vi "UPRcontroller_v00_basedonlsmv66.vi"() -> ()   [LabVIEW 2015] (continued)
                        n4087 = call "tt_timeandsamples.vi"("bin"=w857, "refreshtime"=w851, "srateAODOtt"=w854, "tot#ofsamples"=w859) -> ("refreshrate"=w855:dbl, "refreshbuffer"=w856:i32, "timetracecycles"=w861:i32)  [unwired: 5 in]
                        n4088 = local read "bin"() -> (w858:dbl)
                        n4089 = call "2pparameters.vi"("command"="get") -> ("params out"=w870:T12)  [unwired: 1 in]
                        n4090 = Bundle By Name(cluster=w870, "Drawing Mode"=w843, "measpoints"=w859, "tt_cycles"=w861, "refreshbuffer"=w856, "refreshrate"=w855, "Vx-ref"=w862, "Vy-ref"=w864, "srate"=w853, "finite"=w866, "cont"=w865, "wavdet"=w867, "avpp"=w863, "srateAODO"=w860, "bufferAI"=w856, "bin"=w858, "Angle Img"=w850, "Vxminref"=w849, "Vxmaxref"=w848, "Vyminref"=w847, "Vymaxref"=w846, "Xpixels Img"=w845, "Ypixels Img"=w844, "Pel"=w842, "Vz-reset"=0.0, "AIoverride"=w840, "type"="Timetrace") -> (w868:T12)
                        n4091 = Reciprocal(x=w855) -> (1/x=w852:dbl)
                        n4092 = local write "refreshtime"(w852) -> ()
                        n4093 = call "2pparameters.vi"("Params in"=w868, "command"="set") -> ()  [unwired: 1 out]
                      }
                      frame "Lifetime (point)" {
                      }
                    }
                  }
                  frame #1 {
                    w873 = FALSE ("wavdet")
                    n4094 = call "2pparameters.vi"("command"="get") -> ("params out"=w877:T12)  [unwired: 1 in]
                    n4095 = Bundle By Name(cluster=w877, "finite"=w873, "cont"=w873, "wavdet"=TRUE) -> (w874:T12)
                    n4096 = call "2pparameters.vi"("Params in"=w874, "command"="set") -> ()  [unwired: 1 out]
                  }
                  frame #2 {
                    n4097 = local read "DO channels"() -> (w885:u16)
                    n4098 = call "2pparameters.vi"("command"="get") -> ("params out"=w883:T12)  [unwired: 1 in]
                    n4099 = in-place {
                      in-place-border: w885 -> [w890]
                      in-place-border: [w887] -> w880
                      in-place-border: [w886] -> w879
                      n4100 = in-place-cluster #52(w883) -> ("aDO"=w889:u32[])
                      n4101 = call "remove channel from active arrayv2.vi"("line array in"=w889, "line to remove"=w890) -> ("line array out"=w888:u32[], "removal"=w887:bool, "index"=w886:i32)
                      n4102 = in-place-cluster #52("aDO"=w888) -> (w881:T12)
                    }
                    n4103 = local write "remDO"(w880) -> ()
                    n4104 = call "2pparameters.vi"("Params in"=w881, "command"="set") -> ()  [unwired: 1 out]
                  }
                  frame #3 {
                    n4105 = local read "remDO"() -> (w891:bool)
                    n4106 = case shown="True" w891 {
                      frame False {
                      }
                      frame True {
                        n4107 = call "Used AO lines.vi"() -> ("used AO names"=w895:string[], "used AO lines"=w897:tag[])  [unwired: 2 in]
                        n4108 = local write "Analog Used Lines"(w897) -> ()
                        n4109 = local write "Analog Used Names"(w895) -> ()
                        n4110 = call "Used DO lines.vi"() -> ("used DO names"=w893:string[], "used DO lines"=w892:tag[])  [unwired: 2 in]
                        n4111 = control-ref of="Analog Lines Plot"() -> (w896:refnum<vi>)
                        n4112 = control-ref of="Digital Lines Plot"() -> (w894:refnum<vi>)
                        n4113 = local write "Digital Used Lines"(w892) -> ()
                        n4114 = local write "Digital Used Names"(w893) -> ()
                        n4115 = call "prepAOWaveplot.vi"("WaveformGraph in"=w896, "Analog Used Names"=w895) -> ()  [unwired: 1 in]
                        n4116 = call "prepDOWaveplot.vi"("DigitalGraph in"=w894, "used DO names"=w893) -> ()  [unwired: 1 in]
                      }
                    }
                  }
                  frame #4 {
                    n4117 = local read "remDO"() -> (w899:bool)
                    n4118 = case shown="True" w899 {
                      tunnel: w898 -> [_ w900]
                      frame False {
                      }
                      frame True {
                        n4119 = call "waveformparamsv2.vi"("command"="rem DO", "index"=w900) -> ()  [unwired: 3 in, 3 out]
                      }
                    }
                  }
                  frame #5 {
                    n4120 = local read "Meastab"() -> (w905:enum32{"X-Y Image", "Linescan", "Timetrace"})
                    n4121 = property on="refwf" class="Ring (strict)"() -> ("RingText.Text"=w912:string)  [unwired: 2 in, 2 out]
                    n4122 = call "waveformsDObuffer.vi"("command"="get") -> ("DO wf out"=w911:digitalwaveform[])  [unwired: 1 in]
                    n4123 = case shown="\"Timetrace\"" w905 {
                      tunnel: [w921 w922] -> w904
                      frame "X-Y Image", Default {
                        n4124 = local read "Sampling rate"() -> (w921:dbl)
                      }
                      frame "Timetrace" {
                        n4125 = local read "srateAODOtt"() -> (w922:dbl)
                      }
                    }
                    n4126 = call "waveformsAObuffer.vi"("command"="get") -> ("AO wf out"=w920:waveform(dbl)[])  [unwired: 1 in]
                    n4127 = Delete From Array(array=w911, length=1, index=w909) -> (array with subset deleted=w908:digitalwaveform[])  [unwired: 1 out]
                    n4128 = call "correctwaveformsizetemp.vi"("new sampling frequency (Hz)"=w904, "start"=FALSE, "reference waveforms to"=w912, "Analog waveforms in"=w920, "stop"=FALSE, "Digital waveforms in"=w908) -> ("analog wf out"=w915:waveform(dbl)[], "Digital wf out"=w913:digitalwaveform[], "measpoints"=w906:i32)
                    n4129 = local read "wavdet"() -> (w907:bool)
                    n4130 = call "waveformsAObuffer.vi"("AO wf in"=w915, "command"="set") -> ()  [unwired: 1 out]
                    n4131 = call "waveformsDObuffer.vi"("DO wf in"=w913, "command"="set") -> ()  [unwired: 1 out]
                    n4132 = local write "Analog Lines Plot"(w915) -> ()
                    n4133 = local write "Digital Lines Plot"(w913) -> ()
                    n4134 = call "GetNumCamFramesv2.vi"("Digital Waveform Graph"=w913) -> ("Numeric"=w914:i32)  [unwired: 10 in]
                    n4135 = case shown="True" w907 {
                      tunnel: w906 -> [_ w923]
                      frame False {
                      }
                      frame True {
                        n4136 = local write "# of frames"(w923) -> ()
                      }
                    }
                    n4137 = local write "Total Camera Frames"(w914) -> ()
                  }
                  frame #6 {
                    w924 = FALSE ("addAO")
                    n4138 = local read "finite samples"() -> (w925:bool)
                    n4139 = local read "continuous"() -> (w926:bool)
                    n4140 = local read "wavdet"() -> (w927:bool)
                    n4141 = local write "remDO"(w924) -> ()
                    n4142 = call "2pparameters.vi"("command"="get") -> ("params out"=w930:T12)  [unwired: 1 in]
                    n4143 = Bundle By Name(cluster=w930, "finite"=w925, "cont"=w926, "wavdet"=w927) -> (w928:T12)
                    n4144 = property on="Rem DO wave" class="Bool (strict)"("Val(Sgnl)"=w924) -> ()  [unwired: 2 in, 2 out]
                    n4145 = call "2pparameters.vi"("Params in"=w928, "command"="set") -> ()  [unwired: 1 out]
                  }
                }
              }
            }
          }
          event "load changed DO wave": Value Change {
            n4146 = event-data() -> ("NewVal"=w932:bool)  [unwired: 1 in, 5 out]
            n4147 = case shown="True" w932 {
              frame False {
              }
              frame True {
                n4148 = stacked-sequence {
                  seq-local: [_ _ w1040 _ _] -> [_ _ _ w1057 _]
                  seq-local: [_ _ w1039 _ _] -> [_ _ _ w1056 _]
                  frame #0 {
                    n4149 = local read "Measurement"() -> (w934:T4)
                    n4150 = local write "changeDO"(TRUE ("addAO")) -> ()
                    n4151 = case shown="\"X-Y-t movie\", Default" w934 {
                      frame "X-Y-t movie", Default {
                        n4152 = local read "avpp"() -> (w955:i32)
                        n4153 = local read "Angle ref"() -> (w954:dbl)
                        n4154 = local read "ROI Type"() -> (w953:u16)
                        n4155 = local read "xpixels ref"() -> (w950:i32)
                        n4156 = local read "Vx-min ref"() -> (w949:dbl)
                        n4157 = local read "Vx-max ref"() -> (w948:dbl)
                        n4158 = local read "ypixels ref"() -> (w946:i32)
                        n4159 = local read "Vy-min ref"() -> (w947:dbl)
                        n4160 = local read "Vy-max ref"() -> (w943:dbl)
                        n4161 = local read "Sampling rate"() -> (w937:dbl)
                        n4162 = local read "finite samples"() -> (w938:bool)
                        n4163 = local read "continuous"() -> (w941:bool)
                        n4164 = local read "wavdet"() -> (w942:bool)
                        n4165 = local read "# of frames"() -> (w940:i32)
                        n4166 = local read "maxbufferAI"() -> (w939:i32)
                        n4167 = local read "Override AI buffer"() -> (w935:bool)
                        n4168 = call "2pparameters.vi"("command"="get") -> ("params out"=w952:T12)  [unwired: 1 in]
                        n4169 = Bundle By Name(cluster=w952, "type"="X-Y-t movie", "avpp"=w955, "Angle Img"=w954, "Xpixels Img"=w950, "Vx-min Img"=w949, "VX-max Img"=w948, "Ypixels Img"=w946, "Vy-min Img"=w947, "Vy-max Img"=w943, "srate"=w937, "srate Img"=w937, "finite"=w938, "cont"=w941, "wavdet"=w942, "measpoints"=w940, "maxbufferAI"=w939, "Drawing Mode"=w953, "Vz-reset"=0.0, "AIoverride"=w935) -> (w944:T12)
                        n4170 = call "2pparameters.vi"("Params in"=w944, "command"="set") -> ()  [unwired: 1 out]
                      }
                      frame "X-Y-Z stack" {
                        n4171 = call "2pparameters.vi"("command"="get") -> ("params out"=w959:T12)  [unwired: 1 in]
                        n4172 = Bundle By Name(cluster=w959, "type"="X-Y-Z stack") -> (w957:T12)
                        n4173 = call "2pparameters.vi"("Params in"=w957, "command"="set") -> ()  [unwired: 1 out]
                      }
                      frame "Lifetime (scan)" {
                        n4174 = call "2pparameters.vi"("command"="get") -> ("params out"=w964:T12)  [unwired: 1 in]
                        n4175 = Bundle By Name(cluster=w964, "type"="Lifetime (scan)") -> (w962:T12)
                        n4176 = call "2pparameters.vi"("Params in"=w962, "command"="set") -> ()  [unwired: 1 out]
                      }
                      frame "Lifetime (contour)" {
                        n4177 = local read "Vy-min draw"() -> (w974:dbl)
                        n4178 = local read "Vy-max draw"() -> (w973:dbl)
                        n4179 = local read "Vx-min draw"() -> (w976:dbl)
                        n4180 = local read "Vx-max draw"() -> (w975:dbl)
                        n4181 = local read "xpixels ref"() -> (w972:i32)
                        n4182 = local read "ypixels ref"() -> (w971:i32)
                        n4183 = local read "ROI Type"() -> (w970:u16)
                        n4184 = local read "srateAODOtt"() -> (w981:dbl)
                        n4185 = local read "# of frames"() -> (w986:i32)
                        n4186 = local read "refreshtime"() -> (w978:dbl)
                        n4187 = local read "Pel"() -> (w969:dbl)
                        n4188 = local read "bin"() -> (w984:dbl)
                        n4189 = local read "Override AI buffer"() -> (w967:bool)
                        n4190 = local read "finite samples"() -> (w993:bool)
                        n4191 = local read "srateAODOtt"() -> (w980:dbl)
                        n4192 = local read "srateAODOtt"() -> (w987:dbl)
                        n4193 = local read "continuous"() -> (w992:bool)
                        n4194 = local read "Angle ref"() -> (w977:dbl)
                        n4195 = local read "wavdet"() -> (w994:bool)
                        n4196 = local read "Vx-ref"() -> (w989:dbl)
                        n4197 = local read "Vy-ref"() -> (w991:dbl)
                        n4198 = local read "avpp"() -> (w990:i32)
                        n4199 = call "tt_timeandsamples.vi"("bin"=w984, "refreshtime"=w978, "srateAODOtt"=w981, "tot#ofsamples"=w986) -> ("refreshrate"=w982:dbl, "refreshbuffer"=w983:i32, "timetracecycles"=w988:i32)  [unwired: 5 in]
                        n4200 = local read "bin"() -> (w985:dbl)
                        n4201 = call "2pparameters.vi"("command"="get") -> ("params out"=w997:T12)  [unwired: 1 in]
                        n4202 = Bundle By Name(cluster=w997, "Drawing Mode"=w970, "measpoints"=w986, "tt_cycles"=w988, "refreshbuffer"=w983, "refreshrate"=w982, "Vx-ref"=w989, "Vy-ref"=w991, "srate"=w980, "finite"=w993, "cont"=w992, "wavdet"=w994, "avpp"=w990, "srateAODO"=w987, "bufferAI"=w983, "bin"=w985, "Angle Img"=w977, "Vxminref"=w976, "Vxmaxref"=w975, "Vyminref"=w974, "Vymaxref"=w973, "Xpixels Img"=w972, "Ypixels Img"=w971, "Pel"=w969, "Vz-reset"=0.0, "AIoverride"=w967, "type"="Lifetime (contour)") -> (w995:T12)
                        n4203 = Reciprocal(x=w982) -> (1/x=w979:dbl)
                        n4204 = local write "refreshtime"(w979) -> ()
                        n4205 = call "2pparameters.vi"("Params in"=w995, "command"="set") -> ()  [unwired: 1 out]
                      }
                      frame "X-Y-Z-t movie" {
                      }
                      frame "linescan" {
                      }
                      frame "Timetrace" {
                        n4206 = local read "Vy-min draw"() -> (w1007:dbl)
                        n4207 = local read "Vy-max draw"() -> (w1006:dbl)
                        n4208 = local read "Vx-min draw"() -> (w1009:dbl)
                        n4209 = local read "Vx-max draw"() -> (w1008:dbl)
                        n4210 = local read "xpixels ref"() -> (w1005:i32)
                        n4211 = local read "ypixels ref"() -> (w1004:i32)
                        n4212 = local read "ROI Type"() -> (w1003:u16)
                        n4213 = local read "srateAODOtt"() -> (w1014:dbl)
                        n4214 = local read "# of frames"() -> (w1019:i32)
                        n4215 = local read "refreshtime"() -> (w1011:dbl)
                        n4216 = local read "Pel"() -> (w1002:dbl)
                        n4217 = local read "bin"() -> (w1017:dbl)
                        n4218 = local read "Override AI buffer"() -> (w1000:bool)
                        n4219 = local read "finite samples"() -> (w1026:bool)
                        n4220 = local read "srateAODOtt"() -> (w1013:dbl)
                        n4221 = local read "srateAODOtt"() -> (w1020:dbl)
                        n4222 = local read "continuous"() -> (w1025:bool)
                        n4223 = local read "Angle ref"() -> (w1010:dbl)
                        n4224 = local read "wavdet"() -> (w1027:bool)
                        n4225 = local read "Vx-ref"() -> (w1022:dbl)
                        n4226 = local read "Vy-ref"() -> (w1024:dbl)
                        n4227 = local read "avpp"() -> (w1023:i32)
                        n4228 = call "tt_timeandsamples.vi"("bin"=w1017, "refreshtime"=w1011, "srateAODOtt"=w1014, "tot#ofsamples"=w1019) -> ("refreshrate"=w1015:dbl, "refreshbuffer"=w1016:i32, "timetracecycles"=w1021:i32)  [unwired: 5 in]
                        n4229 = local read "bin"() -> (w1018:dbl)
                        n4230 = call "2pparameters.vi"("command"="get") -> ("params out"=w1030:T12)  [unwired: 1 in]
                        n4231 = Bundle By Name(cluster=w1030, "Drawing Mode"=w1003, "measpoints"=w1019, "tt_cycles"=w1021, "refreshbuffer"=w1016, "refreshrate"=w1015, "Vx-ref"=w1022, "Vy-ref"=w1024, "srate"=w1013, "finite"=w1026, "cont"=w1025, "wavdet"=w1027, "avpp"=w1023, "srateAODO"=w1020, "bufferAI"=w1016, "bin"=w1018, "Angle Img"=w1010, "Vxminref"=w1009, "Vxmaxref"=w1008, "Vyminref"=w1007, "Vymaxref"=w1006, "Xpixels Img"=w1005, "Ypixels Img"=w1004, "Pel"=w1002, "Vz-reset"=0.0, "AIoverride"=w1000, "type"="Timetrace") -> (w1028:T12)
                        n4232 = Reciprocal(x=w1015) -> (1/x=w1012:dbl)
                        n4233 = local write "refreshtime"(w1012) -> ()
                        n4234 = call "2pparameters.vi"("Params in"=w1028, "command"="set") -> ()  [unwired: 1 out]
                      }
                      frame "Lifetime (point)" {
                      }
                    }
                  }
                  frame #1 {
                    w1033 = FALSE ("wavdet")
                    n4235 = call "2pparameters.vi"("command"="get") -> ("params out"=w1037:T12)  [unwired: 1 in]
                    n4236 = Bundle By Name(cluster=w1037, "finite"=w1033, "cont"=w1033, "wavdet"=TRUE) -> (w1034:T12)
                    n4237 = call "2pparameters.vi"("Params in"=w1034, "command"="set") -> ()  [unwired: 1 out]
                  }
                  frame #2 {
                    n4238 = local read "DO channels"() -> (w1042:u16)
                    n4239 = call "2pparameters.vi"("command"="get") -> ("params out"=w1044:T12)  [unwired: 1 in]
                    n4240 = Unbundle By Name(w1044) -> ("aDO"=w1043:u32[])
                    n4241 = Search 1D Array(1D array=w1043, element=w1042) -> (index of element=w1040:i32)  [unwired: 1 in]
                    n4242 = Greater?(x=w1040, y=-1) -> (0:w1039:bool)
                    n4243 = case shown="True" w1039 {
                      tunnel: w1040 -> [_ w1053]
                      frame False {
                      }
                      frame True {
                        n4244 = local read "Meastab"() -> (w1047:enum32{"X-Y Image", "Linescan", "Timetrace"})
                        n4245 = local read "Digital padding value"() -> (w1048:dbl)
                        n4246 = local read "Digital time offset (s)"() -> (w1049:dbl)
                        n4247 = case shown="\"Timetrace\"" w1047 {
                          tunnel: [w1054 w1055] -> w1046
                          frame "X-Y Image", Default {
                            n4248 = local read "Sampling rate"() -> (w1054:dbl)
                          }
                          frame "Timetrace" {
                            n4249 = local read "srateAODOtt"() -> (w1055:dbl)
                          }
                        }
                        n4250 = local read "Digital Freq (Hz)"() -> (w1051:dbl)
                        n4251 = local read "Digital phase (s)"() -> (w1050:dbl)
                        n4252 = local read "Digital DC (%)"() -> (w1052:dbl)
                        n4253 = call "replace DO wf param.vi"("Digital Freq (Hz)"=w1051, "Digital DC (%)"=w1052, "Digital phase"=w1050, "Sampling frequency (Hz)"=w1046, "Digital time offset (s)"=w1049, "index of DO wave"=w1053, "padding value"=w1048) -> ()  [unwired: 4 in]
                      }
                    }
                  }
                  frame #3 {
                    n4254 = case shown="True" w1056 {
                      tunnel: w1057 -> [_ w1064]
                      frame False {
                      }
                      frame True {
                        n4255 = local read "Meastab"() -> (w1061:enum32{"X-Y Image", "Linescan", "Timetrace"})
                        n4256 = call "waveformparamsv2.vi"("command"="get") -> ("Params out"=w1080:T17)  [unwired: 4 in, 2 out]
                        n4257 = Unbundle By Name(w1080) -> ("DO parameters"=w1079:T20)
                        n4258 = property on="refwf" class="Ring (strict)"() -> ("RingText.Text"=w1086:string)  [unwired: 2 in, 2 out]
                        n4259 = case shown="\"Timetrace\"" w1061 {
                          tunnel: [w1087 w1088] -> w1060
                          frame "X-Y Image", Default {
                            n4260 = local read "Sampling rate"() -> (w1087:dbl)
                          }
                          frame "Timetrace" {
                            n4261 = local read "srateAODOtt"() -> (w1088:dbl)
                          }
                        }
                        n4262 = call "waveformsAObuffer.vi"("command"="get") -> ("AO wf out"=w1084:waveform(dbl)[])  [unwired: 1 in]
                        n4263 = call "waveformsDObuffer.vi"("command"="get") -> ("DO wf out"=w1082:digitalwaveform[])  [unwired: 1 in]
                        n4264 = call "referfencesize.vi"("Digital waveforms in"=w1082, "Analog waveforms in"=w1084, "reference waveforms to"=w1086) -> ("number of samples"=w1077:i32)  [unwired: 2 in]
                        n4265 = Index Array(array=w1079, index=w1064) -> (element=w1078:T21)
                        n4266 = call "waveformsDObuffer.vi"("command"="get") -> ("DO wf out"=w1074:digitalwaveform[])  [unwired: 1 in]
                        n4267 = call "simple digital from wf params.vi"("waveform params"=w1078, "number of samples"=w1077) -> ("digital waveform"=w1076:digitalwaveform)
                        n4268 = property on="refwf" class="Ring (strict)"() -> ("RingText.Text"=w1066:string)  [unwired: 2 in, 2 out]
                        n4269 = Replace Array Subset(array=w1074, new element=w1076, index=w1064) -> (w1065:digitalwaveform[])
                        n4270 = call "waveformsAObuffer.vi"("command"="get") -> ("AO wf out"=w1073:waveform(dbl)[])  [unwired: 1 in]
                        n4271 = local read "wavdet"() -> (w1063:bool)
                        n4272 = call "correctwaveformsizetemp.vi"("new sampling frequency (Hz)"=w1060, "start"=FALSE, "reference waveforms to"=w1066, "Analog waveforms in"=w1073, "stop"=FALSE, "Digital waveforms in"=w1065) -> ("analog wf out"=w1069:waveform(dbl)[], "Digital wf out"=w1067:digitalwaveform[], "measpoints"=w1062:i32)
                        n4273 = local write "Analog Lines Plot"(w1069) -> ()
                        n4274 = call "GetNumCamFramesv2.vi"("Digital Waveform Graph"=w1067) -> ("Numeric"=w1068:i32)  [unwired: 10 in]
                        n4275 = local write "Digital Lines Plot"(w1067) -> ()
                        n4276 = case shown="True" w1063 {
                          tunnel: w1062 -> [_ w1089]
                          frame False {
                          }
                          frame True {
                            n4277 = local write "# of frames"(w1089) -> ()
                          }
                        }
                        n4278 = call "waveformsAObuffer.vi"("AO wf in"=w1069, "command"="set") -> ()  [unwired: 1 out]
                        n4279 = call "waveformsDObuffer.vi"("DO wf in"=w1067, "command"="set") -> ()  [unwired: 1 out]
                        n4280 = local write "Total Camera Frames"(w1068) -> ()
                      }
                    }
                  }
                  frame #4 {
                    w1091 = FALSE ("addAO")
                    n4281 = local read "finite samples"() -> (w1092:bool)
                    n4282 = local read "continuous"() -> (w1093:bool)
                    n4283 = local read "wavdet"() -> (w1094:bool)
                    n4284 = local write "changeDO"(w1091) -> ()
                    n4285 = property on="load changed DO wave" class="Bool (strict)"("Val(Sgnl)"=w1091) -> ()  [unwired: 2 in, 2 out]
                    n4286 = call "2pparameters.vi"("command"="get") -> ("params out"=w1097:T12)  [unwired: 1 in]
                    n4287 = Bundle By Name(cluster=w1097, "finite"=w1092, "cont"=w1093, "wavdet"=w1094) -> (w1095:T12)
                    n4288 = local write "not loadedDO"(FALSE ("not loadedDO")) -> ()
                    n4289 = call "2pparameters.vi"("Params in"=w1095, "command"="set") -> ()  [unwired: 1 out]
                  }
                }
              }
            }
          }
          event "refwf": Value Change {
            n4290 = event-data() -> ()  [unwired: 1 in, 6 out]
            n4291 = stacked-sequence {
              frame #0 {
                n4292 = local read "Measurement"() -> (w1099:T4)
                n4293 = case shown="\"Timetrace\"" w1099 {
                  frame "X-Y-t movie", Default {
                    n4294 = local read "avpp"() -> (w1120:i32)
                    n4295 = local read "Angle ref"() -> (w1119:dbl)
                    n4296 = local read "ROI Type"() -> (w1118:u16)
                    n4297 = local read "xpixels ref"() -> (w1115:i32)
                    n4298 = local read "Vx-min ref"() -> (w1114:dbl)
                    n4299 = local read "Vx-max ref"() -> (w1113:dbl)
                    n4300 = local read "ypixels ref"() -> (w1111:i32)
                    n4301 = local read "Vy-min ref"() -> (w1112:dbl)
                    n4302 = local read "Vy-max ref"() -> (w1108:dbl)
                    n4303 = local read "Sampling rate"() -> (w1102:dbl)
                    n4304 = local read "finite samples"() -> (w1103:bool)
                    n4305 = local read "continuous"() -> (w1106:bool)
                    n4306 = local read "wavdet"() -> (w1107:bool)
                    n4307 = local read "# of frames"() -> (w1105:i32)
                    n4308 = local read "maxbufferAI"() -> (w1104:i32)
                    n4309 = local read "Override AI buffer"() -> (w1100:bool)
                    n4310 = call "2pparameters.vi"("command"="get") -> ("params out"=w1117:T12)  [unwired: 1 in]
                    n4311 = Bundle By Name(cluster=w1117, "type"="X-Y-t movie", "avpp"=w1120, "Angle Img"=w1119, "Xpixels Img"=w1115, "Vx-min Img"=w1114, "VX-max Img"=w1113, "Ypixels Img"=w1111, "Vy-min Img"=w1112, "Vy-max Img"=w1108, "srate"=w1102, "srate Img"=w1102, "finite"=w1103, "cont"=w1106, "wavdet"=w1107, "measpoints"=w1105, "maxbufferAI"=w1104, "Drawing Mode"=w1118, "Vz-reset"=0.0, "AIoverride"=w1100) -> (w1109:T12)
                    n4312 = call "2pparameters.vi"("Params in"=w1109, "command"="set") -> ()  [unwired: 1 out]
                  }
                  frame "X-Y-Z stack" {
                    n4313 = call "2pparameters.vi"("command"="get") -> ("params out"=w1124:T12)  [unwired: 1 in]
                    n4314 = Bundle By Name(cluster=w1124, "type"="X-Y-Z stack") -> (w1122:T12)
                    n4315 = call "2pparameters.vi"("Params in"=w1122, "command"="set") -> ()  [unwired: 1 out]
                  }
                  frame "Lifetime (scan)" {
                    n4316 = call "2pparameters.vi"("command"="get") -> ("params out"=w1129:T12)  [unwired: 1 in]
                    n4317 = Bundle By Name(cluster=w1129, "type"="Lifetime (scan)") -> (w1127:T12)
                    n4318 = call "2pparameters.vi"("Params in"=w1127, "command"="set") -> ()  [unwired: 1 out]
                  }
                  frame "Lifetime (contour)" {
                    n4319 = local read "Vy-min draw"() -> (w1139:dbl)
                    n4320 = local read "Vy-max draw"() -> (w1138:dbl)
                    n4321 = local read "Vx-min draw"() -> (w1141:dbl)
                    n4322 = local read "Vx-max draw"() -> (w1140:dbl)
                    n4323 = local read "xpixels ref"() -> (w1137:i32)
                    n4324 = local read "ypixels ref"() -> (w1136:i32)
                    n4325 = local read "ROI Type"() -> (w1135:u16)
                    n4326 = local read "srateAODOtt"() -> (w1146:dbl)
                    n4327 = local read "# of frames"() -> (w1151:i32)
                    n4328 = local read "refreshtime"() -> (w1143:dbl)
                    n4329 = local read "Pel"() -> (w1134:dbl)
                    n4330 = local read "bin"() -> (w1149:dbl)
                    n4331 = local read "Override AI buffer"() -> (w1132:bool)
                    n4332 = local read "finite samples"() -> (w1158:bool)
                    n4333 = local read "srateAODOtt"() -> (w1145:dbl)
                    n4334 = local read "srateAODOtt"() -> (w1152:dbl)
                    n4335 = local read "continuous"() -> (w1157:bool)
                    n4336 = local read "Angle ref"() -> (w1142:dbl)
                    n4337 = local read "wavdet"() -> (w1159:bool)
                    n4338 = local read "Vx-ref"() -> (w1154:dbl)
                    n4339 = local read "Vy-ref"() -> (w1156:dbl)
                    n4340 = local read "avpp"() -> (w1155:i32)
                    n4341 = call "tt_timeandsamples.vi"("bin"=w1149, "refreshtime"=w1143, "srateAODOtt"=w1146, "tot#ofsamples"=w1151) -> ("refreshrate"=w1147:dbl, "refreshbuffer"=w1148:i32, "timetracecycles"=w1153:i32)  [unwired: 5 in]
                    n4342 = local read "bin"() -> (w1150:dbl)
                    n4343 = call "2pparameters.vi"("command"="get") -> ("params out"=w1162:T12)  [unwired: 1 in]
                    n4344 = Bundle By Name(cluster=w1162, "Drawing Mode"=w1135, "measpoints"=w1151, "tt_cycles"=w1153, "refreshbuffer"=w1148, "refreshrate"=w1147, "Vx-ref"=w1154, "Vy-ref"=w1156, "srate"=w1145, "finite"=w1158, "cont"=w1157, "wavdet"=w1159, "avpp"=w1155, "srateAODO"=w1152, "bufferAI"=w1148, "bin"=w1150, "Angle Img"=w1142, "Vxminref"=w1141, "Vxmaxref"=w1140, "Vyminref"=w1139, "Vymaxref"=w1138, "Xpixels Img"=w1137, "Ypixels Img"=w1136, "Pel"=w1134, "Vz-reset"=0.0, "AIoverride"=w1132, "type"="Lifetime (contour)") -> (w1160:T12)
                    n4345 = Reciprocal(x=w1147) -> (1/x=w1144:dbl)
                    n4346 = local write "refreshtime"(w1144) -> ()
                    n4347 = call "2pparameters.vi"("Params in"=w1160, "command"="set") -> ()  [unwired: 1 out]
                  }
                  frame "X-Y-Z-t movie" {
                  }
                  frame "linescan" {
                  }
                  frame "Timetrace" {
                    n4348 = local read "Vy-min draw"() -> (w1172:dbl)
                    n4349 = local read "Vy-max draw"() -> (w1171:dbl)
                    n4350 = local read "Vx-min draw"() -> (w1174:dbl)
                    n4351 = local read "Vx-max draw"() -> (w1173:dbl)
                    n4352 = local read "xpixels ref"() -> (w1170:i32)
                    n4353 = local read "ypixels ref"() -> (w1169:i32)
                    n4354 = local read "ROI Type"() -> (w1168:u16)
                    n4355 = local read "srateAODOtt"() -> (w1179:dbl)
                    n4356 = local read "# of frames"() -> (w1184:i32)
                    n4357 = local read "refreshtime"() -> (w1176:dbl)
                    n4358 = local read "Pel"() -> (w1167:dbl)
                    n4359 = local read "bin"() -> (w1182:dbl)
                    n4360 = local read "Override AI buffer"() -> (w1165:bool)
                    n4361 = local read "finite samples"() -> (w1191:bool)
                    n4362 = local read "srateAODOtt"() -> (w1178:dbl)
                    n4363 = local read "srateAODOtt"() -> (w1185:dbl)
                    n4364 = local read "continuous"() -> (w1190:bool)
                    n4365 = local read "Angle ref"() -> (w1175:dbl)
                    n4366 = local read "wavdet"() -> (w1192:bool)
                    n4367 = local read "Vx-ref"() -> (w1187:dbl)
                    n4368 = local read "Vy-ref"() -> (w1189:dbl)
                    n4369 = local read "avpp"() -> (w1188:i32)
                    n4370 = call "tt_timeandsamples.vi"("bin"=w1182, "refreshtime"=w1176, "srateAODOtt"=w1179, "tot#ofsamples"=w1184) -> ("refreshrate"=w1180:dbl, "refreshbuffer"=w1181:i32, "timetracecycles"=w1186:i32)  [unwired: 5 in]
                    n4371 = local read "bin"() -> (w1183:dbl)
                    n4372 = call "2pparameters.vi"("command"="get") -> ("params out"=w1195:T12)  [unwired: 1 in]
                    n4373 = Bundle By Name(cluster=w1195, "Drawing Mode"=w1168, "measpoints"=w1184, "tt_cycles"=w1186, "refreshbuffer"=w1181, "refreshrate"=w1180, "Vx-ref"=w1187, "Vy-ref"=w1189, "srate"=w1178, "finite"=w1191, "cont"=w1190, "wavdet"=w1192, "avpp"=w1188, "srateAODO"=w1185, "bufferAI"=w1181, "bin"=w1183, "Angle Img"=w1175, "Vxminref"=w1174, "Vxmaxref"=w1173, "Vyminref"=w1172, "Vymaxref"=w1171, "Xpixels Img"=w1170, "Ypixels Img"=w1169, "Pel"=w1167, "Vz-reset"=0.0, "AIoverride"=w1165, "type"="Timetrace") -> (w1193:T12)
                    n4374 = Reciprocal(x=w1180) -> (1/x=w1177:dbl)
                    n4375 = local write "refreshtime"(w1177) -> ()
                    n4376 = call "2pparameters.vi"("Params in"=w1193, "command"="set") -> ()  [unwired: 1 out]
                  }
                  frame "Lifetime (point)" {
                  }
                }
              }
              frame #1 {
                w1198 = FALSE ("wavdet")
                n4377 = call "2pparameters.vi"("command"="get") -> ("params out"=w1202:T12)  [unwired: 1 in]
                n4378 = Bundle By Name(cluster=w1202, "finite"=w1198, "cont"=w1198, "wavdet"=TRUE) -> (w1199:T12)
                n4379 = call "2pparameters.vi"("Params in"=w1199, "command"="set") -> ()  [unwired: 1 out]
              }
              frame #2 {
                n4380 = local read "Meastab"() -> (w1207:enum32{"X-Y Image", "Linescan", "Timetrace"})
                n4381 = property on="refwf" class="Ring (strict)"() -> ("RingText.Text"=w1210:string)  [unwired: 2 in, 2 out]
                n4382 = case shown="\"Timetrace\"" w1207 {
                  tunnel: [w1220 w1221] -> w1206
                  frame "X-Y Image", Default {
                    n4383 = local read "Sampling rate"() -> (w1220:dbl)
                  }
                  frame "Timetrace" {
                    n4384 = local read "srateAODOtt"() -> (w1221:dbl)
                  }
                }
                n4385 = call "waveformsAObuffer.vi"("command"="get") -> ("AO wf out"=w1219:waveform(dbl)[])  [unwired: 1 in]
                n4386 = local read "wavdet"() -> (w1209:bool)
                n4387 = call "waveformsDObuffer.vi"("command"="get") -> ("DO wf out"=w1215:digitalwaveform[])  [unwired: 1 in]
                n4388 = call "correctwaveformsizetemp.vi"("new sampling frequency (Hz)"=w1206, "start"=FALSE, "reference waveforms to"=w1210, "Analog waveforms in"=w1219, "stop"=FALSE, "Digital waveforms in"=w1215) -> ("analog wf out"=w1213:waveform(dbl)[], "Digital wf out"=w1211:digitalwaveform[], "measpoints"=w1208:i32)
                n4389 = local write "Analog Lines Plot"(w1213) -> ()
                n4390 = call "GetNumCamFramesv2.vi"("Digital Waveform Graph"=w1211) -> ("Numeric"=w1212:i32)  [unwired: 10 in]
                n4391 = local write "Digital Lines Plot"(w1211) -> ()
                n4392 = call "waveformsDObuffer.vi"("DO wf in"=w1211, "command"="set") -> ()  [unwired: 1 out]
                n4393 = call "waveformsAObuffer.vi"("AO wf in"=w1213, "command"="set") -> ()  [unwired: 1 out]
                n4394 = local write "Total Camera Frames"(w1212) -> ()
                n4395 = case shown="True" w1209 {
                  tunnel: w1208 -> [_ w1222]
                  frame False {
                  }
                  frame True {
                    n4396 = local write "# of frames"(w1222) -> ()
                  }
                }
              }
              frame #3 {
                n4397 = local read "finite samples"() -> (w1223:bool)
                n4398 = local read "continuous"() -> (w1224:bool)
                n4399 = local read "wavdet"() -> (w1225:bool)
                n4400 = call "2pparameters.vi"("command"="get") -> ("params out"=w1228:T12)  [unwired: 1 in]
                n4401 = Bundle By Name(cluster=w1228, "finite"=w1223, "cont"=w1224, "wavdet"=w1225) -> (w1226:T12)
                n4402 = call "2pparameters.vi"("Params in"=w1226, "command"="set") -> ()  [unwired: 1 out]
              }
            }
          }
          event "load changed AOsq": Value Change {
            n4403 = event-data() -> ("NewVal"=w1230:bool)  [unwired: 1 in, 5 out]
            n4404 = case shown="True" w1230 {
              frame False {
              }
              frame True {
                n4405 = stacked-sequence {
                  seq-local: [_ _ _ w1372 _ _] -> [_ _ _ _ w1397 _]
                  seq-local: [_ _ _ w1371 _ _] -> [_ _ _ _ w1396 _]
                  seq-local: [_ _ w1338 _ _ _] -> [_ _ _ w1370 w1395 w1426]
                  frame #0 {
                    n4406 = local read "Measurement"() -> (w1232:T4)
                    n4407 = local write "changeAOsq"(TRUE ("addAO")) -> ()
                    n4408 = case shown="\"X-Y-t movie\", Default" w1232 {
                      frame "X-Y-t movie", Default {
                        n4409 = local read "avpp"() -> (w1253:i32)
                        n4410 = local read "Angle ref"() -> (w1252:dbl)
                        n4411 = local read "ROI Type"() -> (w1251:u16)
                        n4412 = local read "xpixels ref"() -> (w1248:i32)
                        n4413 = local read "Vx-min ref"() -> (w1247:dbl)
                        n4414 = local read "Vx-max ref"() -> (w1246:dbl)
                        n4415 = local read "ypixels ref"() -> (w1244:i32)
                        n4416 = local read "Vy-min ref"() -> (w1245:dbl)
                        n4417 = local read "Vy-max ref"() -> (w1241:dbl)
                        n4418 = local read "Sampling rate"() -> (w1235:dbl)
                        n4419 = local read "finite samples"() -> (w1236:bool)
                        n4420 = local read "continuous"() -> (w1239:bool)
                        n4421 = local read "wavdet"() -> (w1240:bool)
                        n4422 = local read "# of frames"() -> (w1238:i32)
                        n4423 = local read "maxbufferAI"() -> (w1237:i32)
                        n4424 = local read "Override AI buffer"() -> (w1233:bool)
                        n4425 = call "2pparameters.vi"("command"="get") -> ("params out"=w1250:T12)  [unwired: 1 in]
                        n4426 = Bundle By Name(cluster=w1250, "type"="X-Y-t movie", "avpp"=w1253, "Angle Img"=w1252, "Xpixels Img"=w1248, "Vx-min Img"=w1247, "VX-max Img"=w1246, "Ypixels Img"=w1244, "Vy-min Img"=w1245, "Vy-max Img"=w1241, "srate"=w1235, "srate Img"=w1235, "finite"=w1236, "cont"=w1239, "wavdet"=w1240, "measpoints"=w1238, "maxbufferAI"=w1237, "Drawing Mode"=w1251, "Vz-reset"=0.0, "AIoverride"=w1233) -> (w1242:T12)
                        n4427 = call "2pparameters.vi"("Params in"=w1242, "command"="set") -> ()  [unwired: 1 out]
                      }
                      frame "X-Y-Z stack" {
                        n4428 = call "2pparameters.vi"("command"="get") -> ("params out"=w1257:T12)  [unwired: 1 in]
                        n4429 = Bundle By Name(cluster=w1257, "type"="X-Y-Z stack") -> (w1255:T12)
                        n4430 = call "2pparameters.vi"("Params in"=w1255, "command"="set") -> ()  [unwired: 1 out]
                      }
                      frame "Lifetime (scan)" {
                        n4431 = call "2pparameters.vi"("command"="get") -> ("params out"=w1262:T12)  [unwired: 1 in]
                        n4432 = Bundle By Name(cluster=w1262, "type"="Lifetime (scan)") -> (w1260:T12)
                        n4433 = call "2pparameters.vi"("Params in"=w1260, "command"="set") -> ()  [unwired: 1 out]
                      }
                      frame "Lifetime (contour)" {
                        n4434 = local read "Vy-min draw"() -> (w1272:dbl)
                        n4435 = local read "Vy-max draw"() -> (w1271:dbl)
                        n4436 = local read "Vx-min draw"() -> (w1274:dbl)
                        n4437 = local read "Vx-max draw"() -> (w1273:dbl)
                        n4438 = local read "xpixels ref"() -> (w1270:i32)
                        n4439 = local read "ypixels ref"() -> (w1269:i32)
                        n4440 = local read "ROI Type"() -> (w1268:u16)
                        n4441 = local read "srateAODOtt"() -> (w1279:dbl)
                        n4442 = local read "# of frames"() -> (w1284:i32)
                        n4443 = local read "refreshtime"() -> (w1276:dbl)
                        n4444 = local read "Pel"() -> (w1267:dbl)
                        n4445 = local read "bin"() -> (w1282:dbl)
                        n4446 = local read "Override AI buffer"() -> (w1265:bool)
                        n4447 = local read "finite samples"() -> (w1291:bool)
                        n4448 = local read "srateAODOtt"() -> (w1278:dbl)
                        n4449 = local read "srateAODOtt"() -> (w1285:dbl)
                        n4450 = local read "continuous"() -> (w1290:bool)
                        n4451 = local read "Angle ref"() -> (w1275:dbl)
                        n4452 = local read "wavdet"() -> (w1292:bool)
                        n4453 = local read "Vx-ref"() -> (w1287:dbl)
                        n4454 = local read "Vy-ref"() -> (w1289:dbl)
                        n4455 = local read "avpp"() -> (w1288:i32)
                        n4456 = call "tt_timeandsamples.vi"("bin"=w1282, "refreshtime"=w1276, "srateAODOtt"=w1279, "tot#ofsamples"=w1284) -> ("refreshrate"=w1280:dbl, "refreshbuffer"=w1281:i32, "timetracecycles"=w1286:i32)  [unwired: 5 in]
                        n4457 = local read "bin"() -> (w1283:dbl)
                        n4458 = call "2pparameters.vi"("command"="get") -> ("params out"=w1295:T12)  [unwired: 1 in]
                        n4459 = Bundle By Name(cluster=w1295, "Drawing Mode"=w1268, "measpoints"=w1284, "tt_cycles"=w1286, "refreshbuffer"=w1281, "refreshrate"=w1280, "Vx-ref"=w1287, "Vy-ref"=w1289, "srate"=w1278, "finite"=w1291, "cont"=w1290, "wavdet"=w1292, "avpp"=w1288, "srateAODO"=w1285, "bufferAI"=w1281, "bin"=w1283, "Angle Img"=w1275, "Vxminref"=w1274, "Vxmaxref"=w1273, "Vyminref"=w1272, "Vymaxref"=w1271, "Xpixels Img"=w1270, "Ypixels Img"=w1269, "Pel"=w1267, "Vz-reset"=0.0, "AIoverride"=w1265, "type"="Lifetime (contour)") -> (w1293:T12)
                        n4460 = Reciprocal(x=w1280) -> (1/x=w1277:dbl)
                        n4461 = local write "refreshtime"(w1277) -> ()
                        n4462 = call "2pparameters.vi"("Params in"=w1293, "command"="set") -> ()  [unwired: 1 out]
                      }
                      frame "X-Y-Z-t movie" {
                      }
                      frame "linescan" {
                      }
                      frame "Timetrace" {
                        n4463 = local read "Vy-min draw"() -> (w1305:dbl)
                        n4464 = local read "Vy-max draw"() -> (w1304:dbl)
                        n4465 = local read "Vx-min draw"() -> (w1307:dbl)
                        n4466 = local read "Vx-max draw"() -> (w1306:dbl)
                        n4467 = local read "xpixels ref"() -> (w1303:i32)
                        n4468 = local read "ypixels ref"() -> (w1302:i32)
                        n4469 = local read "ROI Type"() -> (w1301:u16)
                        n4470 = local read "srateAODOtt"() -> (w1312:dbl)
                        n4471 = local read "# of frames"() -> (w1317:i32)
                        n4472 = local read "refreshtime"() -> (w1309:dbl)
                        n4473 = local read "Pel"() -> (w1300:dbl)
                        n4474 = local read "bin"() -> (w1315:dbl)
                        n4475 = local read "Override AI buffer"() -> (w1298:bool)
                        n4476 = local read "finite samples"() -> (w1324:bool)
                        n4477 = local read "srateAODOtt"() -> (w1311:dbl)
                        n4478 = local read "srateAODOtt"() -> (w1318:dbl)
                        n4479 = local read "continuous"() -> (w1323:bool)
                        n4480 = local read "Angle ref"() -> (w1308:dbl)
                        n4481 = local read "wavdet"() -> (w1325:bool)
                        n4482 = local read "Vx-ref"() -> (w1320:dbl)
                        n4483 = local read "Vy-ref"() -> (w1322:dbl)
                        n4484 = local read "avpp"() -> (w1321:i32)
                        n4485 = call "tt_timeandsamples.vi"("bin"=w1315, "refreshtime"=w1309, "srateAODOtt"=w1312, "tot#ofsamples"=w1317) -> ("refreshrate"=w1313:dbl, "refreshbuffer"=w1314:i32, "timetracecycles"=w1319:i32)  [unwired: 5 in]
                        n4486 = local read "bin"() -> (w1316:dbl)
                        n4487 = call "2pparameters.vi"("command"="get") -> ("params out"=w1328:T12)  [unwired: 1 in]
                        n4488 = Bundle By Name(cluster=w1328, "Drawing Mode"=w1301, "measpoints"=w1317, "tt_cycles"=w1319, "refreshbuffer"=w1314, "refreshrate"=w1313, "Vx-ref"=w1320, "Vy-ref"=w1322, "srate"=w1311, "finite"=w1324, "cont"=w1323, "wavdet"=w1325, "avpp"=w1321, "srateAODO"=w1318, "bufferAI"=w1314, "bin"=w1316, "Angle Img"=w1308, "Vxminref"=w1307, "Vxmaxref"=w1306, "Vyminref"=w1305, "Vymaxref"=w1304, "Xpixels Img"=w1303, "Ypixels Img"=w1302, "Pel"=w1300, "Vz-reset"=0.0, "AIoverride"=w1298, "type"="Timetrace") -> (w1326:T12)
                        n4489 = Reciprocal(x=w1313) -> (1/x=w1310:dbl)
                        n4490 = local write "refreshtime"(w1310) -> ()
                        n4491 = call "2pparameters.vi"("Params in"=w1326, "command"="set") -> ()  [unwired: 1 out]
                      }
                      frame "Lifetime (point)" {
                      }
                    }
                  }
                  frame #1 {
                    w1331 = FALSE ("wavdet")
                    n4492 = call "2pparameters.vi"("command"="get") -> ("params out"=w1335:T12)  [unwired: 1 in]
                    n4493 = Bundle By Name(cluster=w1335, "finite"=w1331, "cont"=w1331, "wavdet"=TRUE) -> (w1332:T12)
                    n4494 = call "2pparameters.vi"("Params in"=w1332, "command"="set") -> ()  [unwired: 1 out]
                  }
                  frame #2 {
                    n4495 = local read "Meastab"() -> (w1362:enum32{"X-Y Image", "Linescan", "Timetrace"})
                    n4496 = property on="AO channels" class="Ring (strict)"() -> ("RingText.Text"=w1337:string)  [unwired: 2 in, 2 out]
                    n4497 = property on="refwf" class="Ring (strict)"() -> ("RingText.Text"=w1361:string)  [unwired: 2 in, 2 out]
                    n4498 = local read "Build analog waveform tabs"() -> (w1360:enum32{"Square", "Triangle", "Matlab"})
                    n4499 = case shown="\"X-Y Image\", Default" w1362 {
                      tunnel: [w1368 w1369] -> w1359
                      frame "X-Y Image", Default {
                        n4500 = local read "Sampling rate"() -> (w1368:dbl)
                      }
                      frame "Timetrace" {
                        n4501 = local read "srateAODOtt"() -> (w1369:dbl)
                      }
                    }
                    n4502 = local read "Matlab waveform path"() -> (w1352:path)
                    n4503 = local read "Period (ms)"() -> (w1355:dbl)
                    n4504 = local read "Frequency"() -> (w1354:dbl)
                    n4505 = local read "Tri Repeats"() -> (w1353:dbl)
                    n4506 = local read "Repeats"() -> (w1358:dbl)
                    n4507 = local read "Cycles"() -> (w1357:dbl)
                    n4508 = local read "Pulses"() -> (w1356:dbl)
                    n4509 = call "matlabwfexistsdialogue.vi"("Matlab waveform path"=w1352) -> ("mtalab waveform path out"=w1351:path)
                    n4510 = call "wfsizecalc.vi"("Sampling frequency (Hz)"=w1359, "AOtab"=w1360, "reference waveforms to"=w1361, "channel"=w1337, "Repeats"=w1358, "Cycles"=w1357, "Matlab wave file"=w1351, "pulses"=w1356, "Period (ms)"=w1355, "Frequency"=w1354, "Tri Repeats"=w1353) -> ("total size GB"=w1346:dbl, "gigabytesize wf"=w1342:dbl)  [unwired: 3 in]
                    n4511 = Greater?(x=w1342, y=0.5) -> (0:w1343:bool)
                    n4512 = Number To Fractional String(number=w1342, width (-)=i16 3) -> (F-format string=w1348:string)  [unwired: 2 in]
                    n4513 = Number To Fractional String(number=w1346, width (-)=i16 4) -> (F-format string=w1347:string)  [unwired: 2 in]
                    n4514 = Concatenate Strings("this is a crude approximation:\nyou're about to create a  " ("message"), w1348, " GB waveform for a total of " ("string"), w1347, " GB. Are you sure?" ("string")) -> (w1344:string)
                    n4515 = case shown="True" w1343 {
                      tunnel: w1344 -> [_ w1367]
                      tunnel: [TRUE ("T button?") w1364] -> w1338
                      frame False {
                      }
                      frame True {
                        n4516 = Two Button Dialog(message=w1367, 1:"No, don't do this." ("Center Button Text (\"No\")"), 2:"Yes, continue. " ("Left Button Text (\"Yes\")")) -> (T button?=w1364:bool)
                      }
                    }
                  }
                  frame #3 {
                    n4517 = case shown="True" w1370 {
                      tunnel: [_ w1374] -> w1372
                      tunnel: [_ w1373] -> w1371
                      frame False {
                      }
                      frame True {
                        n4518 = local read "AO channels"() -> (w1376:u32)
                        n4519 = call "2pparameters.vi"("command"="get") -> ("params out"=w1378:T12)  [unwired: 1 in]
                        n4520 = Unbundle By Name(w1378) -> ("aAO"=w1377:u32[])
                        n4521 = Search 1D Array(1D array=w1377, element=w1376) -> (index of element=w1374:i32)  [unwired: 1 in]
                        n4522 = Greater?(x=w1374, y=-1) -> (0:w1373:bool)
                        n4523 = case shown="True" w1373 {
                          tunnel: w1374 -> [_ w1392]
                          frame False {
                          }
                          frame True {
                            n4524 = local read "Meastab"() -> (w1381:enum32{"X-Y Image", "Linescan", "Timetrace"})
                            n4525 = case shown="\"Timetrace\"" w1381 {
                              tunnel: [w1393 w1394] -> w1380
                              frame "X-Y Image", Default {
                                n4526 = local read "Sampling rate"() -> (w1393:dbl)
                              }
                              frame "Timetrace" {
                                n4527 = local read "srateAODOtt"() -> (w1394:dbl)
                              }
                            }
                            n4528 = local read "Start amplitude (V)"() -> (w1389:dbl)
                            n4529 = local read "phase shift (ms)"() -> (w1384:dbl)
                            n4530 = local read "Step size (V)"() -> (w1387:dbl)
                            n4531 = local read "Baseline (V)"() -> (w1388:dbl)
                            n4532 = local read "Period (ms)"() -> (w1385:dbl)
                            n4533 = local read "padding value"() -> (w1382:dbl)
                            n4534 = local read "Repeats"() -> (w1391:dbl)
                            n4535 = local read "Cycles"() -> (w1390:dbl)
                            n4536 = local read "DC (%)"() -> (w1386:dbl)
                            n4537 = local read "Pulses"() -> (w1383:dbl)
                            n4538 = call "replace AO square wf param.vi"("Baseline (V)"=w1388, "Start amplitude (V)"=w1389, "Cycles"=w1390, "Repeats"=w1391, "index of AO wave"=w1392, "Step size (V)"=w1387, "DC (%)"=w1386, "Sampling frequency (Hz)"=w1380, "Period (ms)"=w1385, "Cycle length (s)"=w1384, "Pulses"=w1383, "padding value"=w1382) -> ()  [unwired: 4 in]
                          }
                        }
                      }
                    }
                  }
                  frame #4 {
                    n4539 = case shown="True" w1395 {
                      tunnel: w1397 -> [_ w1399]
                      tunnel: w1396 -> [_ w1398]
                      frame False {
                      }
                      frame True {
                        n4540 = case shown="True" w1398 {
                          tunnel: w1399 -> [_ w1407]
                          frame False {
                          }
                          frame True {
                            n4541 = call "waveformparamsv2.vi"("command"="get") -> ("Params out"=w1421:T17)  [unwired: 4 in, 2 out]
                            n4542 = Unbundle By Name(w1421) -> ("AO parameters"=w1420:T18)
                            n4543 = local read "Meastab"() -> (w1402:enum32{"X-Y Image", "Linescan", "Timetrace"})
                            n4544 = case shown="\"Timetrace\"" w1402 {
                              tunnel: [w1423 w1424] -> w1411
                              frame "X-Y Image", Default {
                                n4545 = local read "Sampling rate"() -> (w1423:dbl)
                              }
                              frame "Timetrace" {
                                n4546 = local read "srateAODOtt"() -> (w1424:dbl)
                              }
                            }
                            n4547 = Index Array(array=w1420, index=w1407) -> (element=w1409:T19)
                            n4548 = call "waveformsAObuffer.vi"("command"="get") -> ("AO wf out"=w1408:waveform(dbl)[])  [unwired: 1 in]
                            n4549 = call "generateRampedSquareWave_fromAOparameters.vi"("AO params"=w1409) -> ("Waveform"=w1406:waveform(dbl))  [unwired: 1 out]
                            n4550 = property on="refwf" class="Ring (strict)"() -> ("RingText.Text"=w1410:string)  [unwired: 2 in, 2 out]
                            n4551 = Replace Array Subset(array=w1408, new element=w1406, index=w1407) -> (w1405:waveform(dbl)[])
                            n4552 = call "waveformsDObuffer.vi"("command"="get") -> ("DO wf out"=w1416:digitalwaveform[])  [unwired: 1 in]
                            n4553 = call "correctwaveformsizetemp.vi"("new sampling frequency (Hz)"=w1411, "start"=FALSE, "reference waveforms to"=w1410, "Analog waveforms in"=w1405, "stop"=FALSE, "Digital waveforms in"=w1416) -> ("analog wf out"=w1414:waveform(dbl)[], "Digital wf out"=w1412:digitalwaveform[], "measpoints"=w1403:i32)
                            n4554 = local read "wavdet"() -> (w1404:bool)
                            n4555 = local write "Analog Lines Plot"(w1414) -> ()
                            n4556 = call "GetNumCamFramesv2.vi"("Digital Waveform Graph"=w1412) -> ("Numeric"=w1413:i32)  [unwired: 10 in]
                            n4557 = local write "Digital Lines Plot"(w1412) -> ()
                            n4558 = call "waveformsAObuffer.vi"("AO wf in"=w1414, "command"="set") -> ()  [unwired: 1 out]
                            n4559 = call "waveformsDObuffer.vi"("DO wf in"=w1412, "command"="set") -> ()  [unwired: 1 out]
                            n4560 = local write "Total Camera Frames"(w1413) -> ()
                            n4561 = case shown="True" w1404 {
                              tunnel: w1403 -> [_ w1425]
                              frame False {
                              }
                              frame True {
                                n4562 = local write "# of frames"(w1425) -> ()
                              }
                            }
                          }
                        }
                      }
                    }
                  }
                  frame #5 {
                    w1427 = FALSE ("addAO")
                    n4563 = local read "finite samples"() -> (w1428:bool)
                    n4564 = local read "continuous"() -> (w1429:bool)
                    n4565 = local read "wavdet"() -> (w1430:bool)
                    n4566 = local write "changeAOsq"(w1427) -> ()
                    n4567 = case shown="True" w1426 {
                      frame False {
                      }
                      frame True {
                        n4568 = local write "not loaded"(FALSE ("not loaded")) -> ()
                      }
                    }
                    n4569 = property on="load changed AOsq" class="Bool (strict)"("Val(Sgnl)"=w1427) -> ()  [unwired: 2 in, 2 out]
                    n4570 = call "2pparameters.vi"("command"="get") -> ("params out"=w1433:T12)  [unwired: 1 in]
                    n4571 = Bundle By Name(cluster=w1433, "finite"=w1428, "cont"=w1429, "wavdet"=w1430) -> (w1431:T12)
                    n4572 = call "2pparameters.vi"("Params in"=w1431, "command"="set") -> ()  [unwired: 1 out]
                  }
                }
              }
            }
          }
          event "load changed AOtri": Value Change {
            n4573 = event-data() -> ("NewVal"=w1436:bool)  [unwired: 1 in, 5 out]
            n4574 = case shown="True" w1436 {
              frame False {
              }
              frame True {
                n4575 = stacked-sequence {
                  seq-local: [_ _ _ w1578 _ _] -> [_ _ _ _ w1599 _]
                  seq-local: [_ _ _ w1577 _ _] -> [_ _ _ _ w1598 _]
                  seq-local: [_ _ w1544 _ _ _] -> [_ _ _ w1576 w1597 w1628]
                  frame #0 {
                    n4576 = local read "Measurement"() -> (w1438:T4)
                    n4577 = local write "changeAOtri"(TRUE ("addAO")) -> ()
                    n4578 = case shown="\"X-Y-t movie\", Default" w1438 {
                      frame "X-Y-t movie", Default {
                        n4579 = local read "avpp"() -> (w1459:i32)
                        n4580 = local read "Angle ref"() -> (w1458:dbl)
                        n4581 = local read "ROI Type"() -> (w1457:u16)
                        n4582 = local read "xpixels ref"() -> (w1454:i32)
                        n4583 = local read "Vx-min ref"() -> (w1453:dbl)
                        n4584 = local read "Vx-max ref"() -> (w1452:dbl)
                        n4585 = local read "ypixels ref"() -> (w1450:i32)
                        n4586 = local read "Vy-min ref"() -> (w1451:dbl)
                        n4587 = local read "Vy-max ref"() -> (w1447:dbl)
                        n4588 = local read "Sampling rate"() -> (w1441:dbl)
                        n4589 = local read "finite samples"() -> (w1442:bool)
                        n4590 = local read "continuous"() -> (w1445:bool)
                        n4591 = local read "wavdet"() -> (w1446:bool)
                        n4592 = local read "# of frames"() -> (w1444:i32)
                        n4593 = local read "maxbufferAI"() -> (w1443:i32)
                        n4594 = local read "Override AI buffer"() -> (w1439:bool)
                        n4595 = call "2pparameters.vi"("command"="get") -> ("params out"=w1456:T12)  [unwired: 1 in]
                        n4596 = Bundle By Name(cluster=w1456, "type"="X-Y-t movie", "avpp"=w1459, "Angle Img"=w1458, "Xpixels Img"=w1454, "Vx-min Img"=w1453, "VX-max Img"=w1452, "Ypixels Img"=w1450, "Vy-min Img"=w1451, "Vy-max Img"=w1447, "srate"=w1441, "srate Img"=w1441, "finite"=w1442, "cont"=w1445, "wavdet"=w1446, "measpoints"=w1444, "maxbufferAI"=w1443, "Drawing Mode"=w1457, "Vz-reset"=0.0, "AIoverride"=w1439) -> (w1448:T12)
                        n4597 = call "2pparameters.vi"("Params in"=w1448, "command"="set") -> ()  [unwired: 1 out]
                      }
                      frame "X-Y-Z stack" {
                        n4598 = call "2pparameters.vi"("command"="get") -> ("params out"=w1463:T12)  [unwired: 1 in]
                        n4599 = Bundle By Name(cluster=w1463, "type"="X-Y-Z stack") -> (w1461:T12)
                        n4600 = call "2pparameters.vi"("Params in"=w1461, "command"="set") -> ()  [unwired: 1 out]
                      }
                      frame "Lifetime (scan)" {
                        n4601 = call "2pparameters.vi"("command"="get") -> ("params out"=w1468:T12)  [unwired: 1 in]
                        n4602 = Bundle By Name(cluster=w1468, "type"="Lifetime (scan)") -> (w1466:T12)
                        n4603 = call "2pparameters.vi"("Params in"=w1466, "command"="set") -> ()  [unwired: 1 out]
                      }
                      frame "Lifetime (contour)" {
                        n4604 = local read "Vy-min draw"() -> (w1478:dbl)
                        n4605 = local read "Vy-max draw"() -> (w1477:dbl)
                        n4606 = local read "Vx-min draw"() -> (w1480:dbl)
                        n4607 = local read "Vx-max draw"() -> (w1479:dbl)
                        n4608 = local read "xpixels ref"() -> (w1476:i32)
                        n4609 = local read "ypixels ref"() -> (w1475:i32)
                        n4610 = local read "ROI Type"() -> (w1474:u16)
                        n4611 = local read "srateAODOtt"() -> (w1485:dbl)
                        n4612 = local read "# of frames"() -> (w1490:i32)
                        n4613 = local read "refreshtime"() -> (w1482:dbl)
                        n4614 = local read "Pel"() -> (w1473:dbl)
                        n4615 = local read "bin"() -> (w1488:dbl)
                        n4616 = local read "Override AI buffer"() -> (w1471:bool)
                        n4617 = local read "finite samples"() -> (w1497:bool)
                        n4618 = local read "srateAODOtt"() -> (w1484:dbl)
                        n4619 = local read "srateAODOtt"() -> (w1491:dbl)
                        n4620 = local read "continuous"() -> (w1496:bool)
                        n4621 = local read "Angle ref"() -> (w1481:dbl)
                        n4622 = local read "wavdet"() -> (w1498:bool)
                        n4623 = local read "Vx-ref"() -> (w1493:dbl)
                        n4624 = local read "Vy-ref"() -> (w1495:dbl)
                        n4625 = local read "avpp"() -> (w1494:i32)
                        n4626 = call "tt_timeandsamples.vi"("bin"=w1488, "refreshtime"=w1482, "srateAODOtt"=w1485, "tot#ofsamples"=w1490) -> ("refreshrate"=w1486:dbl, "refreshbuffer"=w1487:i32, "timetracecycles"=w1492:i32)  [unwired: 5 in]
                        n4627 = local read "bin"() -> (w1489:dbl)
                        n4628 = call "2pparameters.vi"("command"="get") -> ("params out"=w1501:T12)  [unwired: 1 in]
                        n4629 = Bundle By Name(cluster=w1501, "Drawing Mode"=w1474, "measpoints"=w1490, "tt_cycles"=w1492, "refreshbuffer"=w1487, "refreshrate"=w1486, "Vx-ref"=w1493, "Vy-ref"=w1495, "srate"=w1484, "finite"=w1497, "cont"=w1496, "wavdet"=w1498, "avpp"=w1494, "srateAODO"=w1491, "bufferAI"=w1487, "bin"=w1489, "Angle Img"=w1481, "Vxminref"=w1480, "Vxmaxref"=w1479, "Vyminref"=w1478, "Vymaxref"=w1477, "Xpixels Img"=w1476, "Ypixels Img"=w1475, "Pel"=w1473, "Vz-reset"=0.0, "AIoverride"=w1471, "type"="Lifetime (contour)") -> (w1499:T12)
                        n4630 = Reciprocal(x=w1486) -> (1/x=w1483:dbl)
                        n4631 = local write "refreshtime"(w1483) -> ()
                        n4632 = call "2pparameters.vi"("Params in"=w1499, "command"="set") -> ()  [unwired: 1 out]
                      }
                      frame "X-Y-Z-t movie" {
                      }
                      frame "linescan" {
                      }
                      frame "Timetrace" {
                        n4633 = local read "Vy-min draw"() -> (w1511:dbl)
                        n4634 = local read "Vy-max draw"() -> (w1510:dbl)
                        n4635 = local read "Vx-min draw"() -> (w1513:dbl)
                        n4636 = local read "Vx-max draw"() -> (w1512:dbl)
                        n4637 = local read "xpixels ref"() -> (w1509:i32)
                        n4638 = local read "ypixels ref"() -> (w1508:i32)
                        n4639 = local read "ROI Type"() -> (w1507:u16)
                        n4640 = local read "srateAODOtt"() -> (w1518:dbl)
                        n4641 = local read "# of frames"() -> (w1523:i32)
                        n4642 = local read "refreshtime"() -> (w1515:dbl)
                        n4643 = local read "Pel"() -> (w1506:dbl)
                        n4644 = local read "bin"() -> (w1521:dbl)
                        n4645 = local read "Override AI buffer"() -> (w1504:bool)
                        n4646 = local read "finite samples"() -> (w1530:bool)
                        n4647 = local read "srateAODOtt"() -> (w1517:dbl)
                        n4648 = local read "srateAODOtt"() -> (w1524:dbl)
                        n4649 = local read "continuous"() -> (w1529:bool)
                        n4650 = local read "Angle ref"() -> (w1514:dbl)
                        n4651 = local read "wavdet"() -> (w1531:bool)
